vi "set_smith_cursor.vi"(5 "left_center":dbl=300.0, 6 "deco_id":i32, 7 "top_center":dbl=300.0, 8 "vi path":path, 9 "x":dbl, 10 "r":dbl, 11 "show_plot_ref":refnum<vi>) -> ()   [LabVIEW 2025]
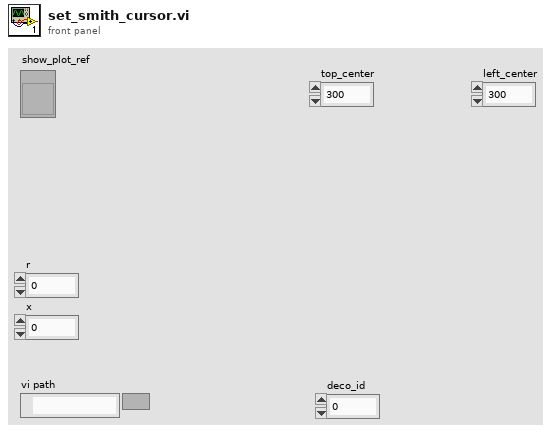
[diagram p1: front panel]
types:
  T1 = typedef "LVPositionTypeDef.ctl" = cluster{"Left":i32, "Top":i32}
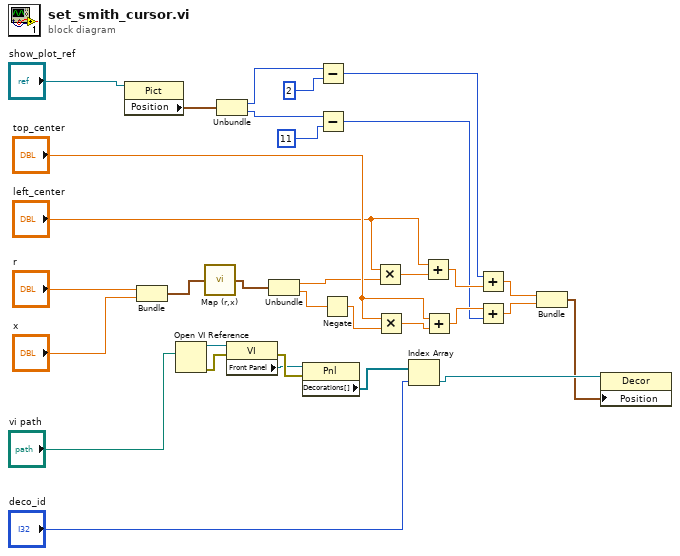
[diagram p0: block diagram]
diagram:
  n1 = property class="Pict"(reference="show_plot_ref") -> ("Position"=w7:T1)  [unwired: 1 in, 2 out]
  n2 = Bundle("r"="r", "x"="x") -> (w30:cluster{"r":dbl, "x":dbl})  [unwired: 1 in]
  n3 = Open VI Reference(vi path="vi path") -> (vi reference=w18:refnum<vi>, error out=w19:errorcluster)  [unwired: 5 in]
  n4 = call <vilib>:"Map (r,x).VI"("Smith Pt"=w30) -> ("Point (h,v)"=w25:cluster{"horizontal":dbl, "vertical":dbl})
  n5 = Unbundle(w7) -> ("Left"=w3:i32, "Top"=w6:i32)
  n6 = property class="VI"(reference=w18, error in=w19) -> (error out=w20:errorcluster, "Front Panel"=w17:refnum<vi>)  [unwired: 1 out]
  n7 = Unbundle(w25) -> ("horizontal"=w24:dbl, "vertical"=w29:dbl)
  n8 = property class="Pnl"(reference=w17, error in=w20) -> ("Decorations[]"=w12:refnum<vi>[])  [unwired: 2 out]
  n9 = Subtract(x=w3, y=2) -> (x-y=w2:i32)
  n10 = Subtract(x=w6, y=11) -> (x-y=w5:i32)
  n11 = Negate(x=w29) -> (-x=w28:dbl)
  n12 = Multiply(x="left_center", y=w24) -> (x*y=w26:dbl)
  n13 = Multiply(x="top_center", y=w28) -> (x*y=w27:dbl)
  n14 = Index Array(array=w12, index="deco_id") -> (element=w21:refnum<vi>)
  n15 = Add(x="left_center", y=w26) -> (x+y=w16:dbl)
  n16 = Add(x="top_center", y=w27) -> (x+y=w15:dbl)
  n17 = Add(x=w2, y=w16) -> (x+y=w14:dbl)
  n18 = Add(x=w15, y=w5) -> (x+y=w13:dbl)
  n19 = Bundle(w14, w13) -> (w10:cluster{dbl, dbl})  [unwired: 1 in]
  n20 = property class="Decor"(reference=w21, "Position"=w10) -> ()  [unwired: 1 in, 2 out]
